vi "chart axis set label position.vi"(8 "error in (no error)":errorcluster, 10 "position":T1 items=["LXW_CHART_AXIS_LABEL_POSITION_NEXT_TO", "LXW_CHART_AXIS_LABEL_POSITION_HIGH", "LXW_CHART_AXIS_LABEL_POSITION_LOW", "LXW_CHART_AXIS_LABEL_POSITION_NONE"], 11 "axis":u32) -> (0 "error out":errorcluster)   [LabVIEW 2015, in "xlsxwriter.lvlib"]
doc: "void chart_axis_set_label_position(lxw_chart_axis axis, uint8_t position);"
uses:
  xlsxwriter.lvlib
  Controls/lxw_chart_axis_label_position.ctl
  xlsxwriter.dll
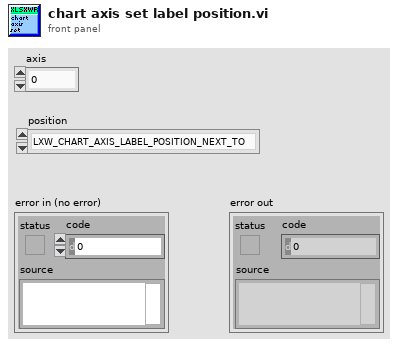
[diagram p1: front panel]
types:
  T1 = typedef "lxw_chart_axis_label_position.ctl" = u8
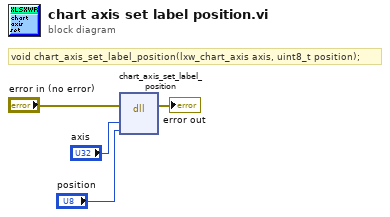
[diagram p0: block diagram]
diagram:
  # "void chart_axis_set_label_position(lxw_chart_axis axis, uint8_t position);"
  n1 = dll-call lib="C:/Users/WDAGUtilityAccount/Desktop/Labview_Example-win32/xlsxwriter.*" fn="chart_axis_set_label_position"(error in="error in (no error)", "axis"="axis", "position"="position") -> (error out=→"error out":errorcluster)  [unwired: 5 in, 1 out]
